vi "FTW-Endpoint-Listen.vi"(0 "FTW Endpoint":refnum<class "FTW-Endpoint.lvclass">, 11 "error in":errorcluster) -> (4 "FTW Endpoint out":refnum<class "FTW-Endpoint.lvclass">, 6 "New Connection":refnum<class "FTW-Endpoint.lvclass">, 15 "error out":errorcluster)   [LabVIEW 2013, in "FTW-Endpoint.lvclass"]
uses:
  FTW-Endpoint.lvclass
  FTW-Endpoint.lvclass/FTW-Endpoint.ctl
panel:
  # "Inputs"
  # "Outputs"
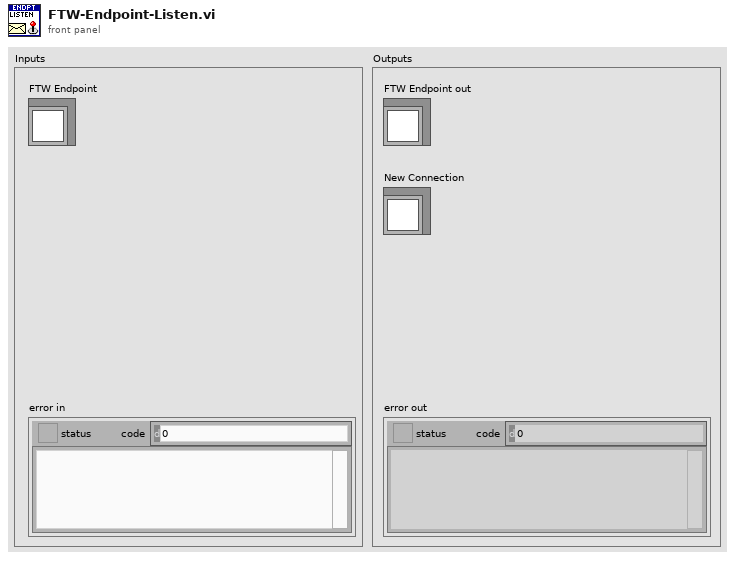
[diagram p1: front panel]
types:
  T1 = typedef "FTW-Message.ctl" = cluster{"Header":string, "Body":string, "Metadata":string}
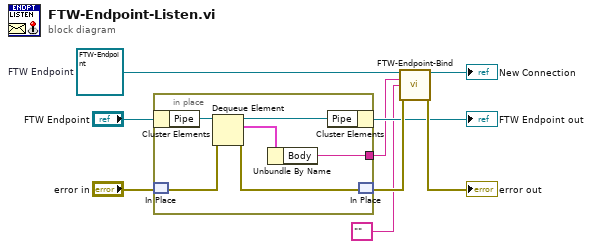
[diagram p0: block diagram]
diagram:
  w4 = refnum<class "FTW-Endpoint.lvclass"> refnum  # FTW Endpoint
  n1 = in-place {
    in-place-border: [w10] -> w2
    n2 = in-place-cluster #1("FTW Endpoint") -> ("Pipe"=w13:refnum<queue>)
    n3 = in-place-match #2("error in") -> (w15:errorcluster)
    n4 = Dequeue Element(queue=w13, error in (no error)=w15) -> (queue out=w12:refnum<queue>, element=w11:T1, error out=w14:errorcluster)  [unwired: 1 in, 1 out]
    n5 = Unbundle By Name(w11) -> ("Body"=w10:string)
    n6 = in-place-cluster #1("Pipe"=w12) -> (→"FTW Endpoint out":refnum<class "FTW-Endpoint.lvclass">)
    n7 = in-place-match #2(w14) -> (w5:errorcluster)
  }
  n8 = call-dynamic "FTW-Endpoint-Bind.vi"("FTW Endpoint"=w4, "Endpoint Address"=w2, "Requested Identity"="", "error in"=w5) -> ("FTW Endpoint out"=→"New Connection":refnum<class "FTW-Endpoint.lvclass">, "error out"=→"error out":errorcluster)  [unwired: 8 in, 2 out]
